vi "Simulation 4.vi"() -> ()   [LabVIEW 2024]
panel:
  out "Encrypted Message Tank 2":dbl
  out "Plain Message Tank 2":dbl
  out "encrypted message Tank 1":dbl
  out "plain message Tank 1":dbl
  out "A2P":bool(c317)
  out "Actuator Valve 2":bool
  out "A1P":bool(c317)
  in  "Actuator Valve 1":bool
  out "Multi-Segment Pipe 5":bool(c317)
  out "A2_pipe":bool(c317)
  out "A1_pipe":bool(c317)
  out "Multi-Segment Pipe 10":bool(c317)
  out "Multi-Segment Pipe 9":bool(c317)
  in  "stop":bool
  in  "Oil Pump":bool
  out "S2":bool
  out "S1":bool
  out "Tank 2":dbl(slide) scale=0.0..100.0
  out "Multi-Segment Pipe 7":bool(c317)
  out "Multi-Segment Pipe 6":bool(c317)
  out "Multi-Segment Pipe 4":bool(c317)
  out "Multi-Segment Pipe 3":bool(c317)
  out "Multi-Segment Pipe 2":bool(c317)
  out "Tank 1":dbl(slide) scale=0.0..100.0
  # "Level Sensor"
  # "Oil Source"
  # "Level Sensor"
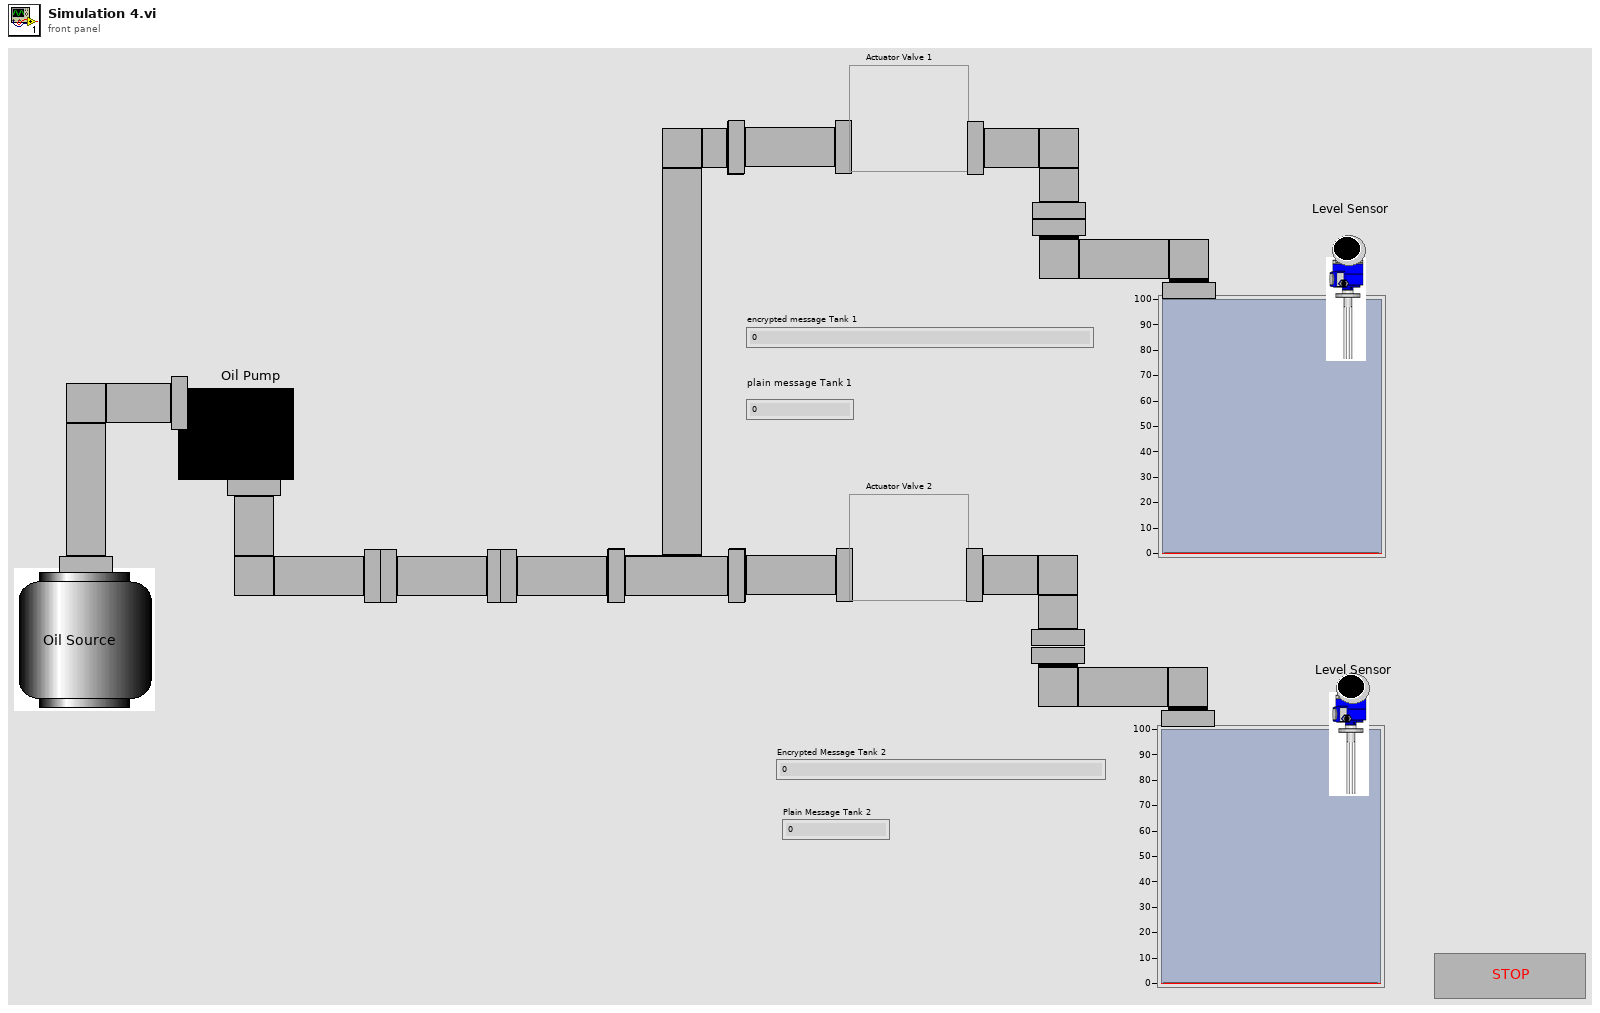
[diagram p1: front panel]
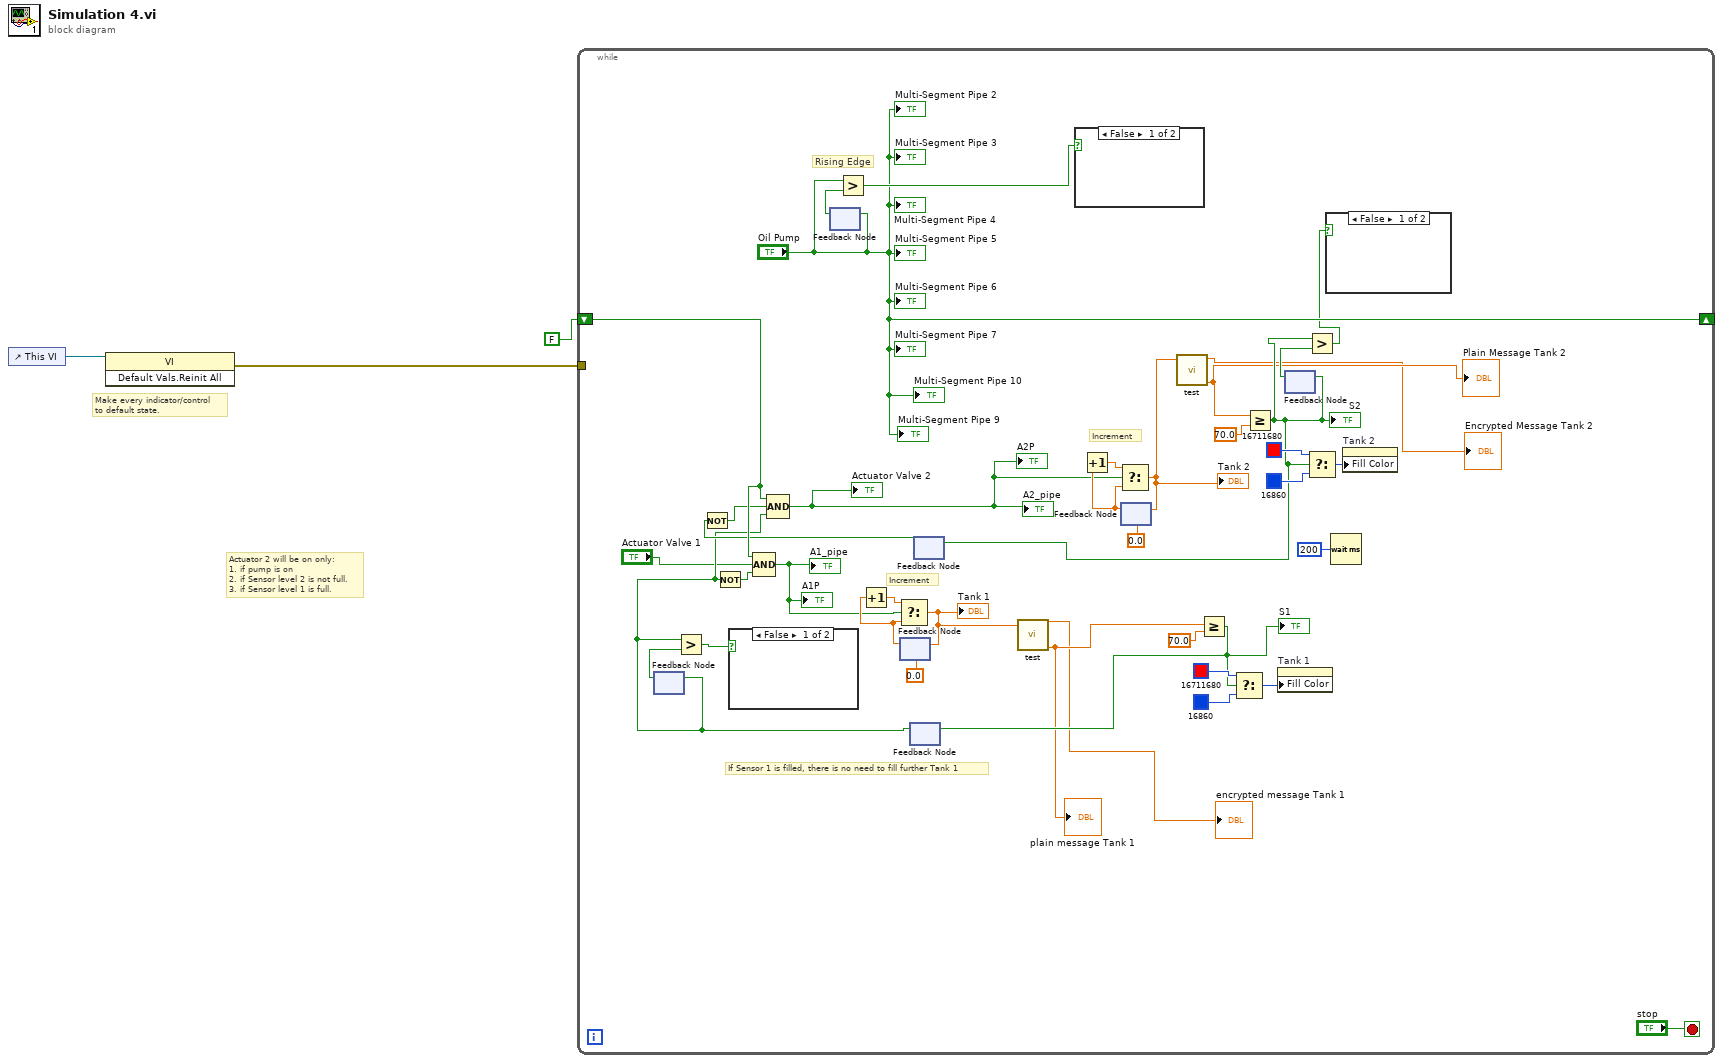
[diagram p0: block diagram]
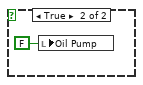
[diagram p2: hidden frame]
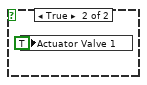
[diagram p3: hidden frame]
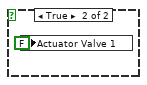
[diagram p4: hidden frame]
diagram:
  # "Actuator 2 will be on only:\n1. if pump is on\n2. if Sensor level 2 is not full.\n3. if Sensor level 1 is full."
  # "Make every indicator/control\nto default state."
  n1 = control-ref of="This VI"() -> (w2:refnum<vi>)
  n2 = invoke class="VI" method="Default Vals.Reinit All"(reference=w2) -> (error out=w1:errorcluster)  [unwired: 2 in, 2 out]
  n3 = while {
    shift-right: ["Oil Pump"] -> _
    shift-left: FALSE -> [w41]
    tunnel: w1 -> [_]
    stop <- "stop" stop-if-true
    # "Increment"
    # "Increment"
    # "If Sensor 1 is filled, there is no need to fill further Tank 1"
    # "Rising Edge"
    n4 = feedback #1() -> (w24:bool)  [unwired: 1 in]
    n5 = feedback #2() -> (w18:bool)  [unwired: 1 in]
    n6 = feedback-in #2("Oil Pump") -> ()
    n7 = Greater?(x="Oil Pump", y=w18) -> (0:w17:bool)
    n8 = feedback #3(0.0) -> (w36:dbl)
    n9 = Increment(x=w36) -> (x+1=w35:dbl)
    n10 = feedback #4() -> (w19:bool)  [unwired: 1 in]
    n11 = feedback-in #1(w19) -> ()
    n12 = Greater?(x=w19, y=w24) -> (0:w23:bool)
    n13 = Not(x=w19) -> (.not. x?=w22:bool)
    n14 = case shown="False" w23 {
      frame False {
      }
      frame True {
        n15 = local write "Actuator Valve 1"(FALSE ("Actuator 1")) -> ()
      }
    }
    n16 = Compound Arithmetic op=AND(w41, "Actuator Valve 1", w22) -> (w12:bool)
    "A1_pipe" <- w12
    "A1P" <- w12
    n17 = Select(t=w35, s=w12, f=w36) -> (s? t:f=w9:dbl)
    "Tank 1" <- w9
    n18 = feedback-in #3(w9) -> ()
    n19 = feedback #5() -> (w21:bool)  [unwired: 1 in]
    n20 = Not(x=w21) -> (.not. x?=w20:bool)
    n21 = Compound Arithmetic op=AND(w41, w20, w19) -> (w10:bool)
    "A2_pipe" <- w10
    "Actuator Valve 2" <- w10
    "A2P" <- w10
    n22 = call "test.vi"("invalue"=w9) -> ("plain message"=w8:dbl, "encrypted Out"=→"encrypted message Tank 1":dbl)  [unwired: 9 in]
    "plain message Tank 1" <- w8
    n23 = case shown="False" w17 {
      frame False {
      }
      frame True {
        n24 = local write "Actuator Valve 1"(TRUE ("Actuator 1")) -> ()
      }
    }
    n25 = feedback #6(0.0) -> (w37:dbl)
    n26 = Increment(x=w37) -> (x+1=w38:dbl)
    n27 = Select(t=w38, s=w10, f=w37) -> (s? t:f=w6:dbl)
    "Tank 2" <- w6
    n28 = feedback-in #6(w6) -> ()
    n29 = call "test.vi"("invalue"=w6) -> ("plain message"=w5:dbl, "encrypted Out"=→"Encrypted Message Tank 2":dbl)  [unwired: 9 in]
    "Plain Message Tank 2" <- w5
    n30 = Greater Or Equal?(x=w8, y=70.0) -> (x >= y?=w25:bool)
    "S1" <- w25
    n31 = feedback-in #4(w25) -> ()
    n32 = Select(t=u32 16711680 ("Fill Color"), s=w25, f=u32 16860 ("Fill Color")) -> (s? t:f=w26:u32)
    n33 = Greater Or Equal?(x=w5, y=70.0) -> (x >= y?=w15:bool)
    "S2" <- w15
    n34 = feedback-in #5(w15) -> ()
    n35 = property on="Tank 1" class="Slide (strict)"("Fill Color"=w26) -> ()  [unwired: 2 in, 2 out]
    n36 = feedback #7() -> (w14:bool)  [unwired: 1 in]
    n37 = feedback-in #7(w15) -> ()
    n38 = Greater?(x=w15, y=w14) -> (0:w13:bool)
    n39 = Select(t=u32 16711680 ("Fill Color"), s=w15, f=u32 16860 ("Fill Color")) -> (s? t:f=w30:u32)
    n40 = case shown="False" w13 {
      frame False {
      }
      frame True {
        n41 = local write "Oil Pump"(FALSE ("Actuator 1")) -> ()
      }
    }
    n42 = Wait (ms)(milliseconds to wait=u32 200) -> ()  [unwired: 1 out]
    n43 = property on="Tank 2" class="Slide (strict)"("Fill Color"=w30) -> ()  [unwired: 2 in, 2 out]
    "Multi-Segment Pipe 2" <- "Oil Pump"
    "Multi-Segment Pipe 3" <- "Oil Pump"
    "Multi-Segment Pipe 4" <- "Oil Pump"
    "Multi-Segment Pipe 5" <- "Oil Pump"
    "Multi-Segment Pipe 6" <- "Oil Pump"
    "Multi-Segment Pipe 7" <- "Oil Pump"
    "Multi-Segment Pipe 9" <- "Oil Pump"
    "Multi-Segment Pipe 10" <- "Oil Pump"
  }
